vi "ELOG_OutputFormat_Get.vi"(8 "error in (no error)":errorcluster, 11 "OXY_SCPI Reseource In":refnum<visa-resource-name>) -> (0 "error out":errorcluster, 1 "communication_data":T1, 2 "Output Format":T2, 3 "OXY_SCPI Reseource Out":refnum<visa-resource-name>)   [LabVIEW 2018, in "OXYGEN.lvlib"]
doc: "Queries the currently configured output format"
uses:
  OXYGEN.lvlib
  TypeDefs/Enum_ELOGOutputFomarts.ctl
  TypeDefs/Cluster_RawCommData.ctl
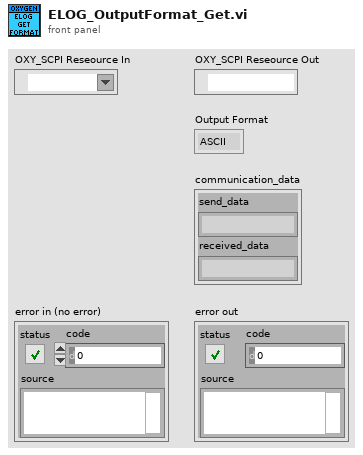
[diagram p1: front panel]
types:
  T1 = typedef "OXYGEN.lvlib/Cluster_RawCommData.ctl" = cluster{"send_data":string, "received_data":string}
  T2 = typedef "OXYGEN.lvlib/Enum_ELOGOutputFomarts.ctl" = enum16{"ASCII", "BIN_INTEL", "BIN_MOTOROLA"}
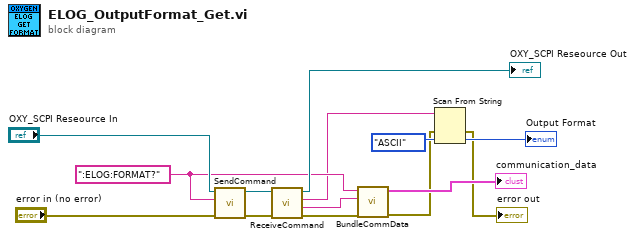
[diagram p0: block diagram]
diagram:
  w4 = ":ELOG:FORMAT?" ("string")
  n1 = call "SendCommand.vi"("error in (no error)"="error in (no error)", "String to Send"=w4, "OXY_SCPI Reseource In"="OXY_SCPI Reseource In") -> ("error out"=w8:errorcluster, "OXY_SCPI Reseource Out"=w9:refnum<visa-resource-name>)  [unwired: 7 in]
  n2 = call "ReceiveCommand.vi"("error in (no error)"=w8, "OXY_SCPI Reseource In"=w9) -> ("error out"=w6:errorcluster, "received Data with Header"=w5:string, "received Data"=w3:string, "OXY_SCPI Reseource Out"=→"OXY_SCPI Reseource Out":refnum<visa-resource-name>)  [unwired: 6 in]
  n3 = call "BundleCommData.vi"("error in (no error)"=w6, "received_data"=w5, "send_data"=w4) -> ("error out"=w2:errorcluster, "communication_data"=→"communication_data":T1)  [unwired: 7 in]
  n4 = Scan From String "Scan From String"(input string=w3, error in=w2, default 1=Enum_ELOGOutputFomarts."ASCII" ("Output Format 2")) -> (error out=→"error out":errorcluster, output 1=→"Output Format":T2)  [unwired: 2 in, 2 out]
